vi "TimeInterpPose2d_GetNewestSample.vi"(11 "TimeInterpPose2d":T1 {"Pose"."ROTATION"."SIN" format="%13.4f"; "Pose"."ROTATION"."COS" format="%13.4f"; "Pose"."ROTATION"."VALUE" format="%13.4f"; "Pose"."TRANSLATION"."Y" format="%14.3f"; "Pose"."TRANSLATION"."X" format="%14.3f"}) -> (1 "IsPresent":bool, 2 "TimeStamp":dbl, 3 "OutputPose2d":T2={"TRANSLATION"={"X"=0.0, "Y"=0.0}, "ROTATION"={"VALUE"=0.0, "COS"=1.0, "SIN"=0.0}} {"ROTATION"."SIN" format="%13.4f"; "ROTATION"."COS" format="%13.4f"; "ROTATION"."VALUE" format="%13.4f"; "TRANSLATION"."Y" format="%14.3f"; "TRANSLATION"."X" format="%14.3f"})   [LabVIEW 2019, in "Trajectory_Library.lvlib"]
doc: "Get the newest sample\n\nInputs:\n - TimeInterpPose2d -- Input data cluster\n\nOutputs\n - OutputPose2d -- Newest Pose2d. \n - TimeStamp -- Time for this sample (seconds)\n - IsPresent -- Returns TRUE if the buffer contains any data"
uses:
  Trajectory_Library.lvlib
  TypeDef/POSE2D.ctl
  TypeDef/TRANSLATION2D.ctl
  TypeDef/ROTATION2D.ctl
  TypeDef/TIME_INTERPOLATABLE_POSE2D.ctl
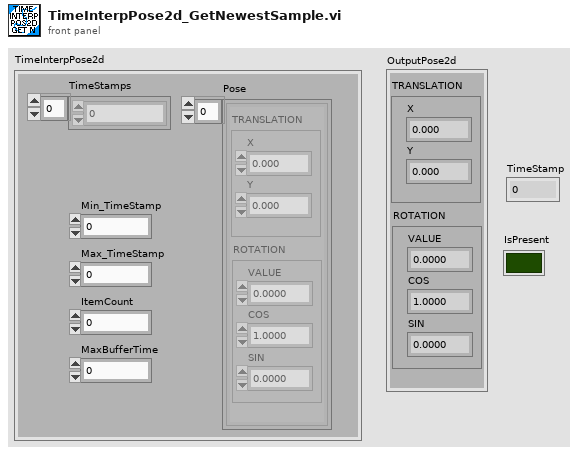
[diagram p1: front panel]
types:
  T1 = typedef "Trajectory_Library.lvlib/TIME_INTERPOLATABLE_POSE2D.ctl" = cluster{"TimeStamps":dbl[], "Pose":T2[], "Min_TimeStamp":dbl, "Max_TimeStamp":dbl, "ItemCount":i32, "MaxBufferTime":dbl}
  T2 = typedef "Trajectory_Library.lvlib/POSE2D.ctl" = cluster{"TRANSLATION":T3, "ROTATION":T4}
  T3 = typedef "Trajectory_Library.lvlib/TRANSLATION2D.ctl" = cluster{"X":dbl, "Y":dbl}
  T4 = typedef "Trajectory_Library.lvlib/ROTATION2D.ctl" = cluster{"VALUE":dbl, "COS":dbl, "SIN":dbl}
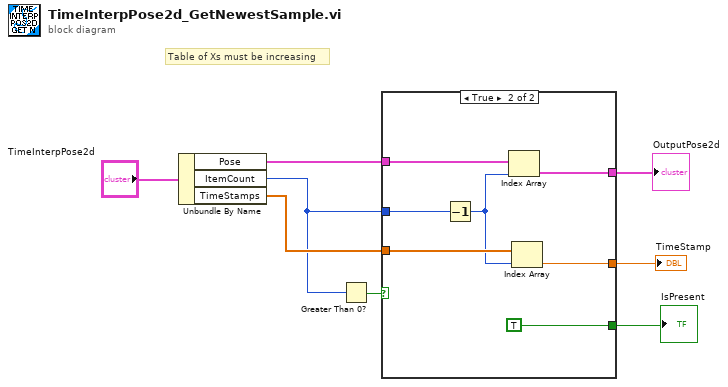
[diagram p0: block diagram]
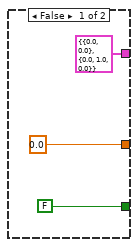
[diagram p2: hidden frame]
diagram:
  # "Table of Xs must be increasing"
  n1 = Unbundle By Name("TimeInterpPose2d") -> ("Pose"=w6:T2[], "ItemCount"=w4:i32, "TimeStamps"=w7:dbl[])
  n2 = Greater Than 0?(x=w4) -> (x > 0?=w5:bool)
  n3 = case shown="True" w5 {
    tunnel: [T2 {"TRANSLATION"={"X"=0.0, "Y"=0.0}, "ROTATION"={"VALUE"=0.0, "COS"=1.0, "SIN"=0.0}} ("Table Y") w15] -> w2
    tunnel: w4 -> [_ w13]
    tunnel: w7 -> [_ w17]
    tunnel: w6 -> [_ w18]
    tunnel: [FALSE TRUE] -> w3
    tunnel: [0.0 w16] -> w1
    frame False {
    }
    frame True {
      n4 = Decrement(x=w13) -> (x-1=w12:i32)
      n5 = Index Array(array=w18, index=w12) -> (element=w15:T2)
      n6 = Index Array(array=w17, index=w12) -> (element=w16:dbl)
    }
  }
  "OutputPose2d" <- w2
  "IsPresent" <- w3
  "TimeStamp" <- w1
